vi "HoodSetpointSelect.vi"(4 "HoodManualControlActive":bool, 5 "ManualSetpointEnable":bool, 7 "ManualSetpointActivate":bool, 8 "VisionTarget":T1, 9 "HoodAutoAimAngle":dbl, 10 "AutoTargetActivate":bool, 11 "ManualSetpoint(deg)":dbl) -> (1 "Setpoint(deg)":dbl, 2 "ActivateAutoControl":bool)   [LabVIEW 2019]
uses:
  Vision/TypeDefs/VisionTarget.ctl
  ArgosLib/Signal Processing/TypeDefs/EdgeDetector_Type.ctl
  ArgosLib/ArgosLib.lvlib
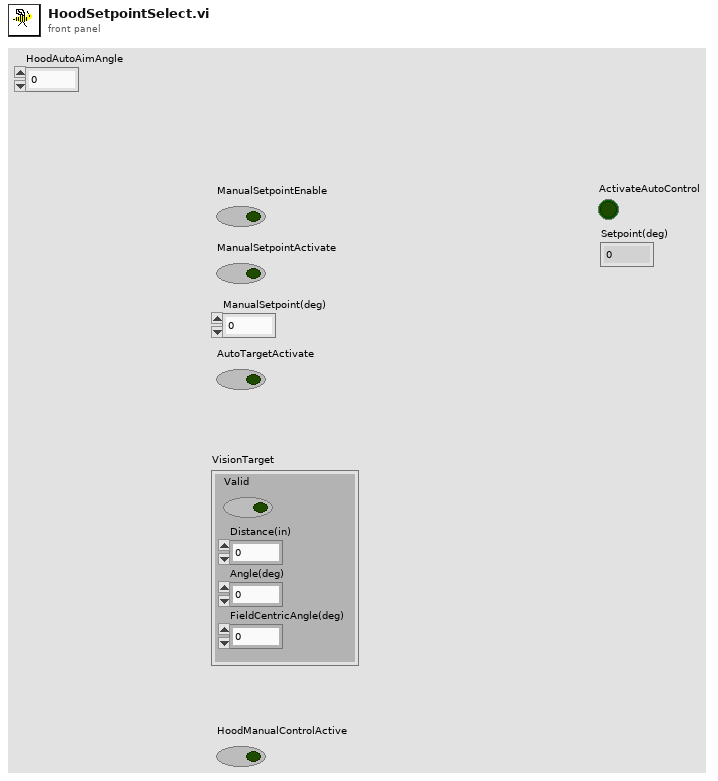
[diagram p1: front panel]
types:
  T1 = typedef "VisionTarget.ctl" = cluster{"Valid":bool, "Distance(in)":dbl, "Angle(deg)":dbl, "FieldCentricAngle(deg)":dbl}
  T2 = typedef "ArgosLib.lvlib/EdgeDetector_Type.ctl" = enum16{"RisingEdge", "FallingEdge", "Both"}
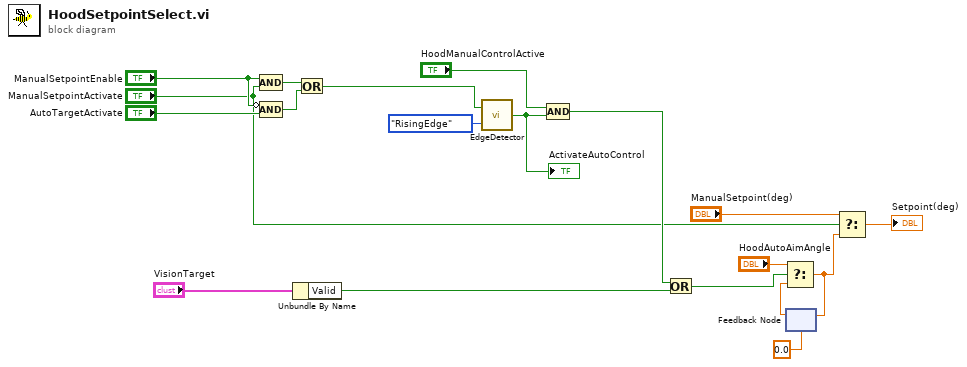
[diagram p0: block diagram]
diagram:
  n1 = Compound Arithmetic op=AND("ManualSetpointEnable", "ManualSetpointActivate") -> (w18:bool)
  n2 = Compound Arithmetic op=AND(invert "ManualSetpointEnable", "AutoTargetActivate") -> (w17:bool)
  n3 = Unbundle By Name("VisionTarget") -> ("Valid"=w7:bool)
  n4 = Or(x=w18, y=w17) -> (x .or. y?=w16:bool)
  n5 = call "EdgeDetector.vi"("DetectorType"=EdgeDetector_Type."RisingEdge", "Input"=w16) -> ("Edge"=w2:bool)
  "ActivateAutoControl" <- w2
  n6 = Compound Arithmetic op=AND("HoodManualControlActive", w2) -> (w8:bool)
  n7 = Or(x=w8, y=w7) -> (x .or. y?=w9:bool)
  n8 = feedback #1(0.0) -> (w11:dbl)
  n9 = Select(t="HoodAutoAimAngle", s=w9, f=w11) -> (s? t:f=w10:dbl)
  n10 = feedback-in #1(w10) -> ()
  n11 = Select(t="ManualSetpoint(deg)", s="ManualSetpointActivate", f=w10) -> (s? t:f=→"Setpoint(deg)":dbl)
